vi "Put Signal.vi"(0 "Connection in":refnum<class "Connection.lvclass">, 5 "Data":refnum<class "Data.lvclass">, 7 "Time":refnum<class "Data.lvclass">, 9 "Path in":string, 11 "error in (no error)":errorcluster) -> (4 "Connection out":refnum<class "Connection.lvclass">, 15 "error out":errorcluster)   [LabVIEW 2015, in "MDSplus.lvlib" / "Connection.lvclass"]
uses:
  Connection.lvclass
  Data_Class/Data.lvclass
  Connection.lvclass/Connection.ctl
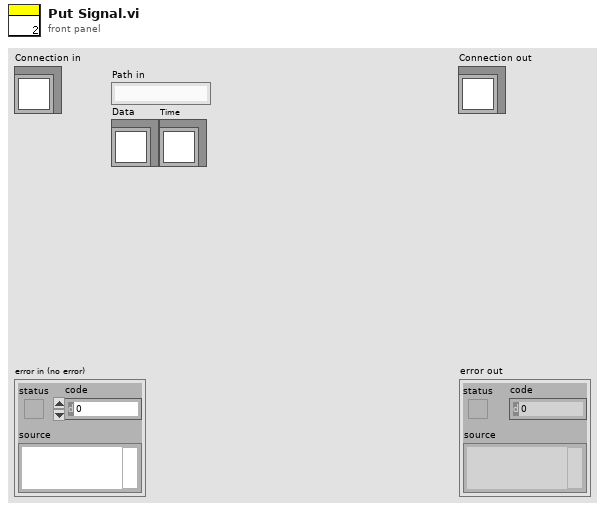
[diagram p1: front panel]
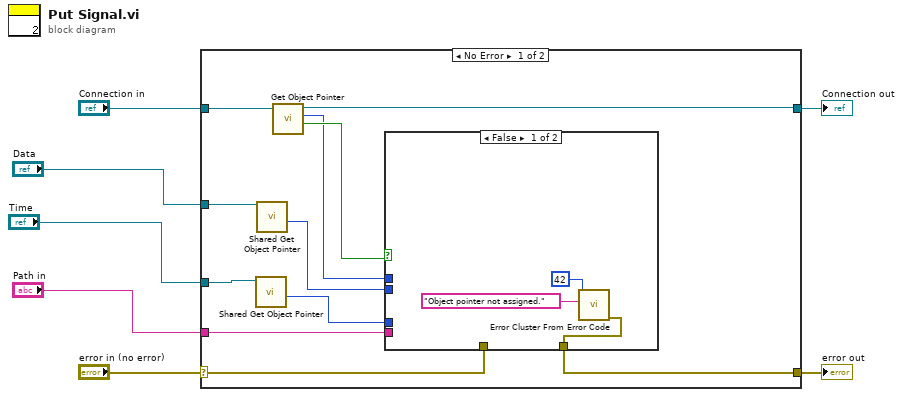
[diagram p0: block diagram]
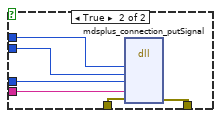
[diagram p2: hidden frame]
diagram:
  n1 = case shown="No Error" "error in (no error)" {
    selector: "error in (no error)" -> [w9 w29]
    tunnel: [w8 w29] -> w6
    tunnel: [w14 w28] -> w4
    tunnel: "Connection in" -> [w15 w28]
    tunnel: "Data" -> [w13 _]
    tunnel: "Time" -> [w12 _]
    tunnel: "Path in" -> [w10 _]
    frame No Error {
      n2 = call "Shared Get Object Pointer.vi"("Data in"=w12) -> ("Object Pointer"=w17:i64)  [unwired: 8 in, 2 out]
      n3 = call "Shared Get Object Pointer.vi"("Data in"=w13) -> ("Object Pointer"=w11:i64)  [unwired: 8 in, 2 out]
      n4 = call "Get Object Pointer.vi"("Connection in"=w15) -> ("Assigned object pointer?"=w18:bool, "Object Pointer"=w16:i64, "Connection out"=w14:refnum<class "Connection.lvclass">)  [unwired: 7 in, 1 out]
      n5 = case shown="False" w18 {
        tunnel: w17 -> [_ w26]
        tunnel: w16 -> [_ w27]
        tunnel: w11 -> [_ w25]
        tunnel: w10 -> [_ w24]
        tunnel: w9 -> [_ w23]
        tunnel: [w19 w22] -> w8
        frame False {
          n6 = call <vilib>:"Error Cluster From Error Code.vi"("error message (\"\")"="Object pointer not assigned." ("error message (\"\")"), "error code (0)"=42) -> ("error out"=w19:errorcluster)  [unwired: 7 in]
        }
        frame True {
          n7 = dll-call lib="MDSobjectsLVShr" fn="mdsplus_connection_putSignal"("lvConnection"=w27, "lvDataPtrIn"=w25, "lvTimePtrIn"=w26, "pathIn"=w24, w23) -> (w22:errorcluster)  [unwired: 8 in, 2 out]
        }
      }
    }
    frame Error {
    }
  }
  "error out" <- w6
  "Connection out" <- w4
